vi "Async VI Control_Write HW Inputs.vi"(8 "error in":errorcluster, 10 "Hardware Output FIFO":refnum<k33>, 11 "Channel Pairs":T3 {"Block Data Refs"."Data Reference" format="%.0x"}) -> (0 "error out":errorcluster, 2 "Write Occured":bool, 3 "Channel Pairs":T3 {"Block Data Refs"."Data Reference" format="%.0x"})   [LabVIEW 2013, in "CANOpen Addon Custom Device.lvlib"]
uses:
  CANOpen Addon Custom Device.lvlib
  <vilib>/NI Veristand/Custom Device API/Block Data Reference.ctl
  <vilib>/NI Veristand/Custom Device API/Data Reference.ctl
  <vilib>/NI Veristand/Custom Device API/Global Data Refs.vi
  <vilib>/NI Veristand/Custom Device API/Custom Device API.lvlib
  Debug/SubVIs/Global debug.vi
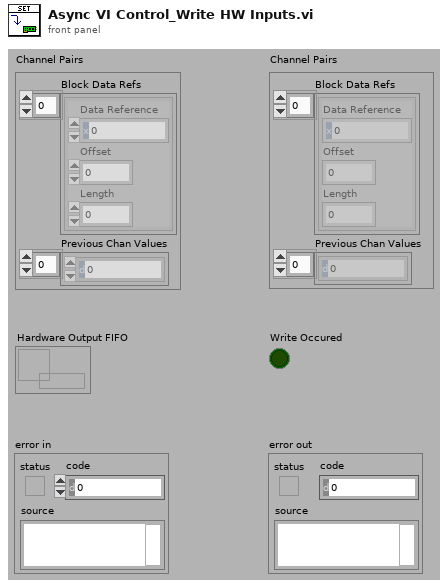
[diagram p1: front panel]
types:
  T1 = typedef "Custom Device API.lvlib/Block Data Reference.ctl" = cluster{"Data Reference":T2, "Offset":i32, "Length":i32}
  T2 = typedef "Custom Device API.lvlib/Data Reference.ctl" = i32
  T3 = cluster{"Block Data Refs":T1[], "Previous Chan Values":dbl[]}
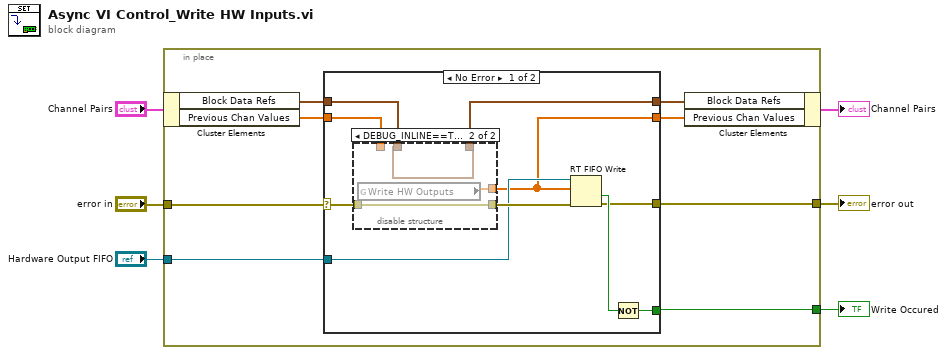
[diagram p0: block diagram]
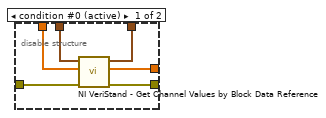
[diagram p2: hidden frame]
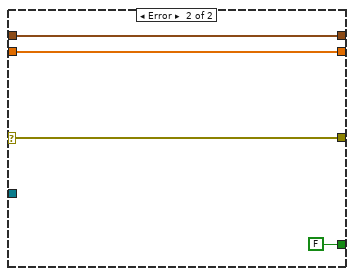
[diagram p3: hidden frame]
diagram:
  n1 = in-place {
    in-place-border: [w14] -> w6
    in-place-border: [w13] -> w5
    in-place-border: "error in" -> [w10]
    in-place-border: "Hardware Output FIFO" -> [w7]
    n2 = in-place-cluster #1("Channel Pairs") -> ("Block Data Refs"=w12:T1[], "Previous Chan Values"=w9:dbl[])
    n3 = case shown="No Error" w10 {
      selector: w10 -> [w21 w37]
      tunnel: [w22 w37] -> w14
      tunnel: [w15 w34] -> w8
      tunnel: [w23 FALSE ("C Read Occured?")] -> w13
      tunnel: w12 -> [w19 w35]
      tunnel: [w18 w35] -> w11
      tunnel: w9 -> [w17 w34]
      tunnel: w7 -> [w16 _]
      frame No Error {
        n4 = disable-structure shown="DEBUG_INLINE==TRUE" {
          disable-tunnel: w21 -> [w30 w33]
          disable-tunnel: [w29 w33] -> w20
          disable-tunnel: w19 -> [w28 w32]
          disable-tunnel: [w27 w32] -> w18
          disable-tunnel: w17 -> [w26 _]
          disable-tunnel: [w25 w31] -> w15
          frame condition #0 (active) {
            n5 = call <vilib>:"NI VeriStand - Get Channel Values by Block Data Reference.vi"("error in (no error)"=w30, "Values Array in"=w26, "Block Data Ref"=w28) -> ("error out"=w29:errorcluster, "Values Array out"=w25:dbl[], "Block Data Ref dup"=w27:T1[])  [unwired: 6 in]
          }
          frame condition #1 {
            n6 = global read "Global debug.vi" "Write HW Outputs"() -> (w31:dbl[])
          }
        }
        n7 = RT FIFO Write(0:w16, 1:w15, 3:w20) -> (10:w24:bool, 11:w22:errorcluster)  [unwired: 2 in, 2 out]
        n8 = Not(x=w24) -> (.not. x?=w23:bool)
      }
      frame Error {
      }
    }
    n9 = in-place-cluster #1("Block Data Refs"=w11, "Previous Chan Values"=w8) -> (→"Channel Pairs":T3)
  }
  "error out" <- w6
  "Write Occured" <- w5
